vi "TwoCodes.vi"(8 "VI Name":string, 10 "Backpack":T1, 11 "Spike":T1) -> ()   [LabVIEW 2019]
uses:
  <userlib>/MicroPython/VIs/uPythonX/uPythonX.xctl
panel:
  in  "main.py":T1(xcontrol)
  in  "Load Libraries":bool
  in  "main.py":T1(xcontrol)
  # "SPIKE Prime"
  # "Backpack"
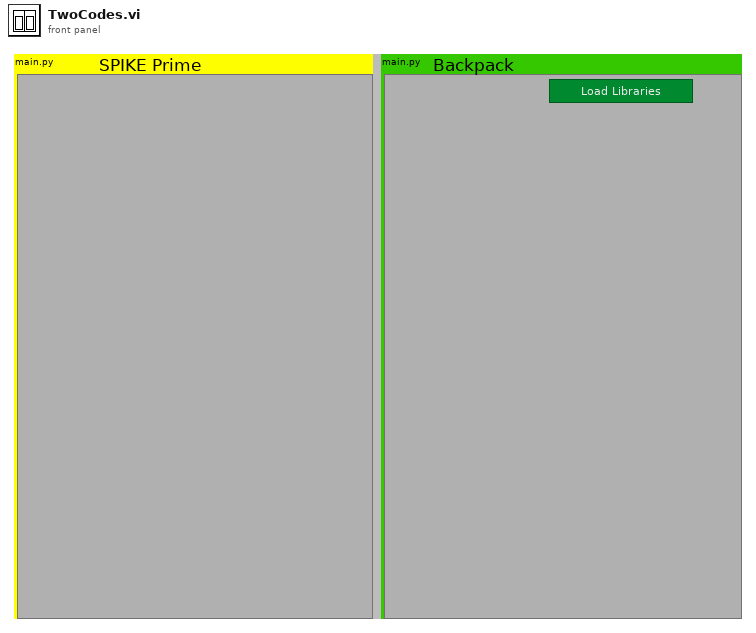
[diagram p1: front panel]
types:
  T1 = cluster{"Port":refnum<visa-resource-name>, "All Code":string}
  T2 = cluster{"Port":refnum<visa-resource-name>, string}
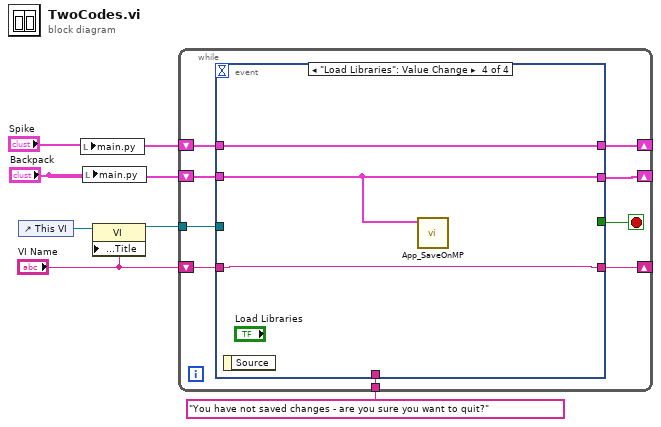
[diagram p0: block diagram]
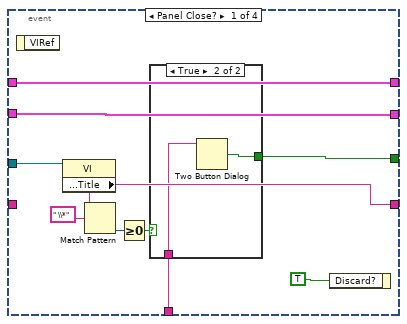
[diagram p2: hidden frame]
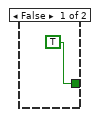
[diagram p3: hidden frame]
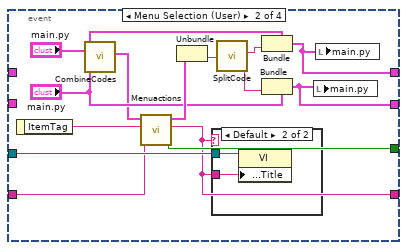
[diagram p4: hidden frame]
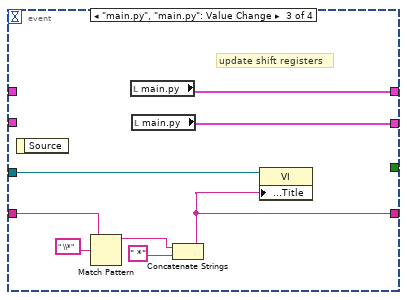
[diagram p6: hidden frame]
diagram:
  n1 = control-ref of="This VI"() -> (w6:refnum<vi>)
  n2 = local write "main.py"("Spike") -> ()
  n3 = local write "main.py"("Backpack") -> ()
  n4 = property class="VI"(reference=w6, "Front Panel.Title"="VI Name") -> (reference out=w5:refnum<vi>)  [unwired: 1 in, 1 out]
  n5 = while {
    tunnel: w5 -> [w14]
    tunnel: "You have not saved changes - are you sure you want to quit?" ("message") -> [w13]
    shift-right: [w12] -> _
    shift-left: "Spike" -> [w11]
    shift-right: [w10] -> _
    shift-left: "Backpack" -> [w9]
    shift-right: [w7] -> _
    shift-left: "VI Name" -> [w8]
    stop <- w15 stop-if-true
    n6 = event shown="[3] \"Load Libraries\": Value Change" {
      selector: _ -> [_ _ _ _]
      dyn-events: _ -> [_ _ _ _]
      timeout: _ -> [_ _ _ _]
      tunnel: [w21 w40 _ _] -> w15
      tunnel: w14 -> [w20 w41 w49 _]
      tunnel: w13 -> [w19 _ _ _]
      tunnel: [w18 w34 w46 w54] -> w12
      tunnel: w11 -> [w18 _ _ w54]
      tunnel: [w17 w32 w45 w53] -> w10
      tunnel: w9 -> [w17 _ _ w53]
      tunnel: w8 -> [_ w39 w48 w55]
      tunnel: [w16 w38 w47 w55] -> w7
      event Panel Close? {
        n7 = event-data() -> ()  [unwired: 1 in, 1 out]
        n8 = property class="VI"(reference=w20) -> ("Front Panel.Title"=w16:string)  [unwired: 1 in, 2 out]
        n9 = Match Pattern(string=w16, regular expression=" \\*" ("string")) -> (offset past match=w24:i32)  [unwired: 1 in, 3 out]
        n10 = Greater Or Equal To 0?(x=w24) -> (x >= 0?=w23:bool)
        n11 = case shown="True" w23 {
          tunnel: [TRUE ("T button?") w28] -> w21
          tunnel: w19 -> [_ w27]
          frame False {
          }
          frame True {
            n12 = Two Button Dialog(message=w27) -> (T button?=w28:bool)  [unwired: 2 in]
          }
        }
        n13 = event-data("Discard?"=TRUE) -> ()  [unwired: 1 in, 1 out]
      }
      event Menu Selection (User) {
        n14 = event-data() -> ("ItemTag"=w42:string)  [unwired: 1 in]
        n15 = call <userlib>:"CombineCodes.vi"("BP Main"="main.py", "Spike Main"="main.py") -> ("Combined"=w29:T2)  [unwired: 9 in]
        n16 = call <userlib>:"Menuactions.vi"("Name"=w39, "ItemTag"=w42, "Default in"=w29) -> ("Close?"=w40:bool, "Name out"=w38:string, "Default out"=w37:T1)  [unwired: 6 in]
        n17 = Unbundle(w37) -> ("All Code"=w36:string)  [unwired: 1 out]
        n18 = case shown="Default" w38 {
          tunnel: w41 -> [_ w44]
          tunnel: w38 -> [_ w43]
          frame "" {
          }
          frame Default {
            n19 = property class="VI"(reference=w44, "Front Panel.Title"=w43) -> ()  [unwired: 1 in, 2 out]
          }
        }
        n20 = call <userlib>:"SplitCode.vi"("Code"=w36) -> ("BP Code"=w33:string, "Spike Code"=w35:string)  [unwired: 9 in]
        n21 = Bundle(cluster="main.py", "All Code"=w35) -> (w34:T1)  [unwired: 1 in]
        n22 = Bundle(cluster="main.py", "All Code"=w33) -> (w32:T1)  [unwired: 1 in]
        n23 = local write "main.py"(w32) -> ()
        n24 = local write "main.py"(w34) -> ()
      }
      event "main.py", "main.py": Value Change {
        # "update shift registers"
        n25 = event-data() -> ()  [unwired: 1 in, 1 out]
        n26 = Match Pattern(string=w48, regular expression=" \\*" ("string")) -> (before substring=w50:string)  [unwired: 1 in, 3 out]
        n27 = local read "main.py"() -> (w46:T1)
        n28 = local read "main.py"() -> (w45:T1)
        n29 = Concatenate Strings(w50, " *" ("string")) -> (w47:string)
        n30 = property class="VI"(reference=w49, "Front Panel.Title"=w47) -> ()  [unwired: 1 in, 2 out]
      }
      event "Load Libraries": Value Change {
        n31 = event-data() -> ()  [unwired: 1 in, 1 out]
        n32 = call <userlib>:"App_SaveOnMP.vi"("Spike"=w53) -> ()  [unwired: 11 in]
      }
    }
  }
